vi "InfoFile2ExpNum.vi"(11 "File Paths":T1={"Local Save Path"=path "\\\\smbhome.uscs.susx.ac.uk\\cv222/Desktop/data", "Newton Save Path"=path "Z:/#Projects/Entanglement/data", "File Name"="test", "LocalSave"=TRUE}) -> (3 "ExpNum string":string)   [LabVIEW 2019]
uses:
  controls/FilePaths.ctl
  controls/GlobalExp.vi
  Global.lvlib
panel:
  in  "Array":cluster{"ExpNum":dbl, "ExpType":string}[](array[cluster]) {"ExpNum" format="%_3f"}
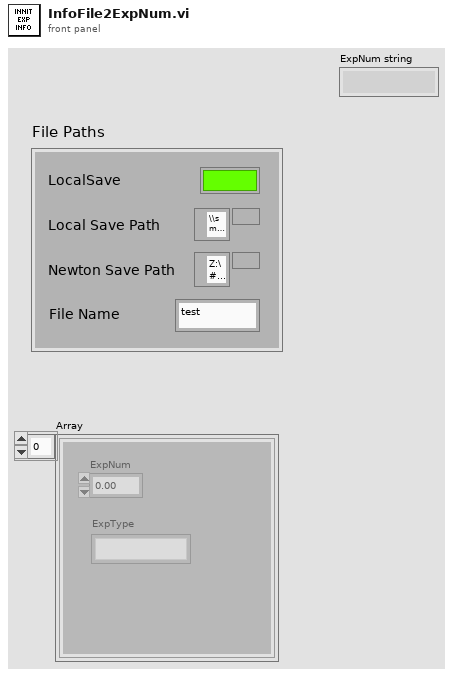
[diagram p1: front panel]
types:
  T1 = typedef "FilePaths.ctl" = cluster{"Local Save Path":path, "Newton Save Path":path, "File Name":string, "LocalSave":bool}
  T2 = enum16{"open", "replace", "create", "open or create", "replace or create", "replace or create with confirmation"}
  T3 = typedef "MasterExpControl.ctl" = cluster{"Main Steps":dbl, "Main Runs":dbl, "ExpStatus":enum16{"Innit", "Stop", "Idle", "MainRunning", "AuxRunning"}, "Main Current Step":dbl, "ExpNum":dbl, "NewData":bool, "date":string, "command":string, "Stop":bool, "Pause":bool, "Mathematica":string, "Main/Meta":bool, "UpdateMath":bool, "Camera":bool, "MetaExpOver":bool, "NextMetaExp":bool}
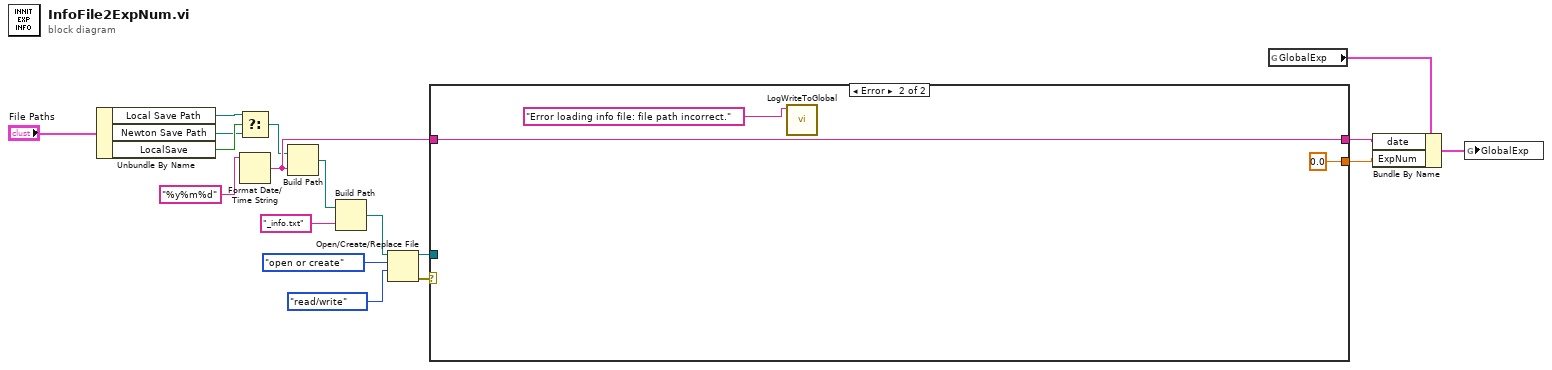
[diagram p0: block diagram]
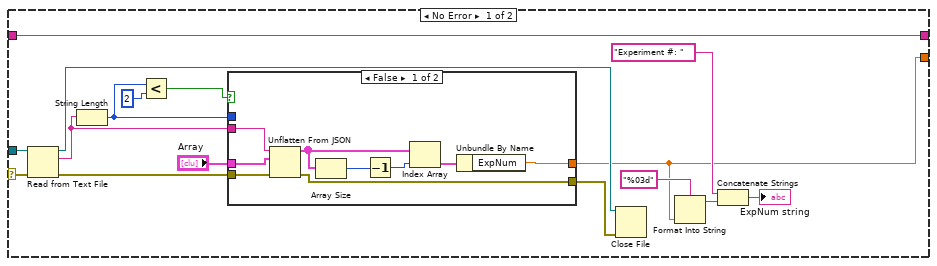
[diagram p2: hidden frame]
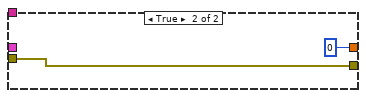
[diagram p3: hidden frame]
diagram:
  n1 = Unbundle By Name("File Paths") -> ("Local Save Path"=w15:path, "Newton Save Path"=w14:path, "LocalSave"=w16:bool)
  n2 = Select(t=w15, s=w16, f=w14) -> (s? t:f=w7:path)
  n3 = Format Date/Time String(time format string (%c)="%y%m%d") -> (date/time string=w13:string)  [unwired: 2 in]
  n4 = Build Path(base path=w7, name or relative path=w13) -> (appended path=w6:path)
  n5 = Build Path(base path=w6, name or relative path="_info.txt") -> (appended path=w11:path)
  n6 = Open/Create/Replace File(file path (use dialog)=w11, operation (0:open)=T2."open or create", access (0:read/write)=enum16{"read/write", "read-only", "write-only"}."read/write") -> (refnum out=w8:refnum<file>, error out=w1:errorcluster)  [unwired: 3 in, 1 out]
  n7 = case shown="Error" w1 {
    selector: w1 -> [w19 _]
    tunnel: w13 -> [w21 w47]
    tunnel: w8 -> [w34 _]
    tunnel: [w21 w47] -> w3
    tunnel: [w20 0.0 ("ExpNum")] -> w2
    frame No Error {
      n8 = Read from Text File(file (use dialog)=w34, error in=w19) -> (refnum out=w33:refnum<file>, text=w25:string, error out=w22:errorcluster)  [unwired: 2 in, 1 out]
      n9 = String Length(string=w25) -> (length=w26:i32)
      n10 = Less?(x=w26, y=2) -> (x < y?=w32:bool)
      n11 = case shown="False" w32 {
        tunnel: [w41 i16 0 ("ExpNum")] -> w20
        tunnel: w26 -> [_ _]
        tunnel: w25 -> [w40 _]
        tunnel: "Array" -> [w39 _]
        tunnel: [w38 w44] -> w23
        tunnel: w22 -> [w37 w44]
        frame False {
          n12 = Unflatten From JSON(JSON string=w40, type and defaults=w39, error in (no error)=w37) -> (value=w36:cluster{"ExpNum":dbl, "ExpType":string}[], error out=w38:errorcluster)  [unwired: 4 in]
          n13 = Array Size(array=w36) -> (size(s)=w35:i32)
          n14 = Decrement(x=w35) -> (x-1=w43:i32)
          n15 = Index Array(array=w36, index=w43) -> (element=w42:cluster{"ExpNum":dbl, "ExpType":string})
          n16 = Unbundle By Name(w42) -> ("ExpNum"=w41:dbl)
        }
        frame True {
        }
      }
      n17 = Close File(refnum=w33, error in=w23) -> ()  [unwired: 2 out]
      n18 = Format Into String(format string="%03d", w20) -> (resulting string=w28:string)  [unwired: 2 in, 1 out]
      n19 = Concatenate Strings("Experiment #: " ("string"), w28) -> (→"ExpNum string":string)
    }
    frame Error {
      n20 = call "LogWriteToGlobal.vi"("in string"="Error loading info file: file path incorrect.") -> ()  [unwired: 11 in]
    }
  }
  n21 = global read "GlobalExp.vi" "GlobalExp"() -> (w4:T3)
  n22 = Bundle By Name(cluster=w4, "date"=w3, "ExpNum"=w2) -> (w5:T3)
  n23 = global write "GlobalExp.vi" "GlobalExp"(w5) -> ()
